vi "SubVI_Classificador_de_cor.vi"(8 "error in":errorcluster, 9 "ROI Objeto":T3 {"Contours"."Type" items=["No Selection", "Point", "Line", "Rectangle", "Oval", "Polygon", "Free", "Annulus", "Unused2", "Unused3", "Broken Line", "Free Hand Line", "Rotated Rectangle"]}, 10 "Classifier Session":T2, 11 "Session In":T1) -> (0 "error out":errorcluster, 2 "Class":string, 3 "Session Out":T1)   [LabVIEW 2017]
uses:
  <vilib>/userdefined/High Color/IMAQdx.ctl
  <vilib>/vision/Classification.llb/IMAQ Classifier Session.ctl
  <vilib>/vision/driver/IMAQdx.llb/IMAQdx Buffer Number Mode.ctl
  <vilib>/vision/driver/NI_Vision_Acquisition_Software.lvlib
  <vilib>/vision/NI_Vision_Development_Module.lvlib
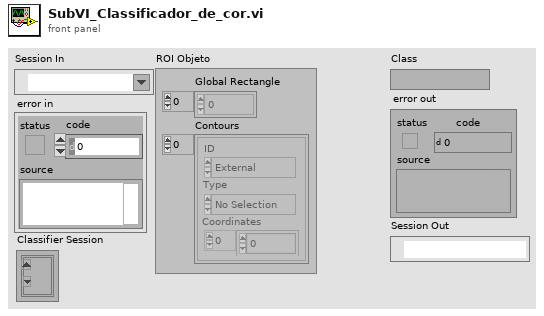
[diagram p1: front panel]
types:
  T1 = typedef "IMAQdx.ctl" = refnum<k21>
  T2 = typedef "IMAQ Classifier Session.ctl" = refnum<k1>
  T3 = cluster{"Global Rectangle":i32[], "Contours":cluster{"ID":enum32{"External", "Internal"}, "Type":u32, "Coordinates":i32[]}[]}
  T4 = typedef "NI_Vision_Acquisition_Software.lvlib/IMAQdx Buffer Number Mode.ctl" = enum32{"Next", "Last", "Buffer Number", "Every", "Last New"}
  T5 = typedef "IMAQ Image.ctl" = refnum<image>
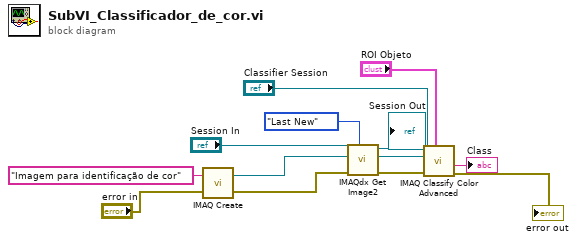
[diagram p0: block diagram]
diagram:
  n1 = call "IMAQ Create"("Image Name"="Imagem para identificação de cor", "error in (no error)"="error in") -> ("New Image"=w11:T5, "error out"=w4:errorcluster)  [unwired: 3 in]
  n2 = call <vilib>:"IMAQdx Get Image2.vi"("Buffer Number Mode (Next)"=IMAQdx_Buffer_Number_Mode."Last New", "error in"=w4, "Image In"=w11, "Session In"="Session In") -> ("error out"=w3:errorcluster, "Image Out"=w9:T5, "Session Out"=→"Session Out":T1)  [unwired: 4 in, 1 out]
  n3 = call "IMAQ Classify Color Advanced"("ROI Descriptor"="ROI Objeto", "error in (no error)"=w3, "Image"=w9, "Classifier Session"="Classifier Session") -> ("error out"=→"error out":errorcluster, "Class"=→"Class":string)  [unwired: 6 out]
